vi "Do Scoring Async.vi"(11 "Submission LLB":path) -> (0 "error out":errorcluster, 2 "Test Summary":string, 3 "Score":T1)   [LabVIEW 2020, in "SOL-Scorer.lvlib"]
uses:
  SOL-Scorer.lvlib
  SoL Scoring/Score.ctl
  SoL Scoring/Score Entry.ctl
  SoL Scoring/SoL Scoring.lvlib
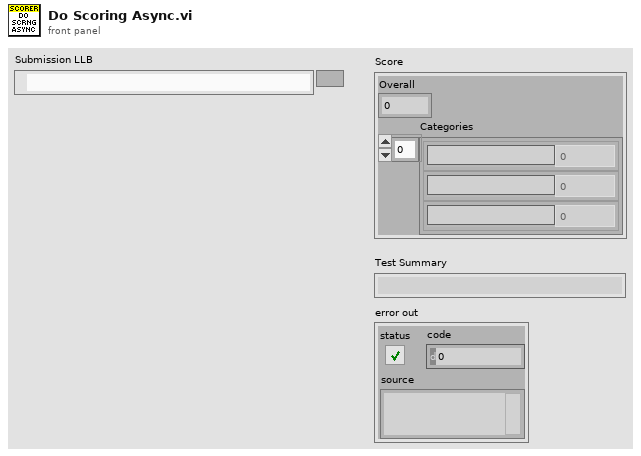
[diagram p1: front panel]
types:
  T1 = typedef "SoL Scoring.lvlib/Score.ctl" = cluster{"Overall":dbl, "Categories":T2[]}
  T2 = typedef "SoL Scoring.lvlib/Score Entry.ctl" = cluster{"Category":string, "Value":dbl}
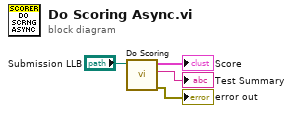
[diagram p0: block diagram]
diagram:
  n1 = call "Do Scoring.vi"("Submission LLB"="Submission LLB") -> ("error out"=→"error out":errorcluster, "Test Summary"=→"Test Summary":string, "Score"=→"Score":T1)  [unwired: 8 in]
